vi "Log Alarm.vi"(8 "error in (no error)":errorcluster, 11 "Message":string) -> (0 "error out":errorcluster)   [LabVIEW 2020, in "Logger Actor API.lvclass"]
uses:
  Logger Actor API.lvclass
  Base Actor/API/Actor API.lvclass
  Global Framework References.vi
  C:/dev/PGS/2001 - TBCM/Source/RT/RTAF/Source/RTAF/Actors/Base Actor/API/Actor API.lvclass
  C:/dev/PGS/2001 - TBCM/Source/RT/RTAF/Source/RTAF/Actors/Logger/API/Logger Actor API.lvclass
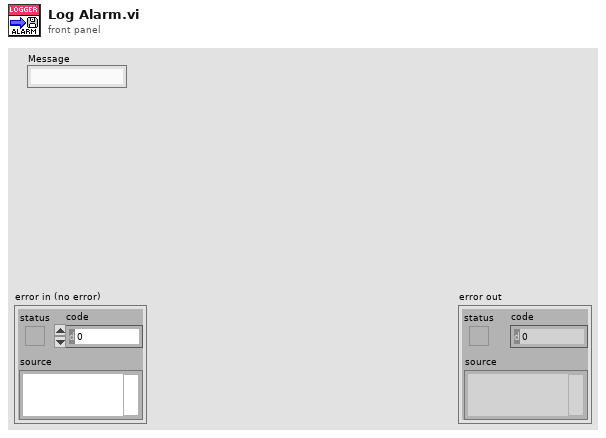
[diagram p1: front panel]
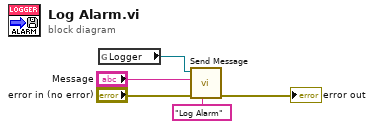
[diagram p0: block diagram]
diagram:
  n1 = global read "Global Framework References.vi" "Logger"() -> (w1:refnum<class "Logger Actor API.lvclass">)
  n2 = call "Send Message.vi"("Name"="Log Alarm", "error in (no error)"="error in (no error)", "Payload"="Message", "Actor API in"=w1) -> ("error out"=→"error out":errorcluster)  [unwired: 7 in]
